vi "parseILC.vi"(8 "error in (no error)":errorcluster, 9 "Func":u8=255, 10 "ModbusBuffer in":refnum<class "ModbusBuffer.lvclass">, 11 "ILC in":refnum<class "ILC.lvclass">) -> (0 "error out":errorcluster, 1 "ParseSuccessful":bool, 2 "ModbusBuffer out":refnum<class "ModbusBuffer.lvclass">, 3 "ILC out":refnum<class "ILC.lvclass">)   [LabVIEW 2016, in "RTILC.lvlib" / "ILC.lvclass"]
uses:
  ILC.lvclass
  Common_RT_Modbus/ModbusBuffer/ModbusBuffer.lvclass
  Common_RT_Modbus/ModbusBuffer/ModbusBuffer.lvclass/ModbusBuffer.ctl
  ILC.lvclass/ILC.ctl
  Common_RT_Modbus/ModbusBuffer/calculateCRC.vi
  Common_RT_Modbus/ModbusBuffer/readCRC.vi
  Common_RT_Modbus/ModbusBuffer/readTimestamp.vi
  Common_RT_Modbus/ModbusBuffer/readEndOfFrame.vi
  Common_RT_Modbus/ModbusBuffer/readU48.vi
  Common_RT_Modbus/ModbusBuffer/readString.vi
  Common_RT_Modbus/ModbusBuffer/readU16.vi
  Common_RT_Modbus/ModbusBuffer/readSGL.vi
  Common_RT_Modbus/ModbusBuffer/readInstructionByte.vi
  Common_RT_Modbus/ModbusBuffer/readTimestampByte.vi
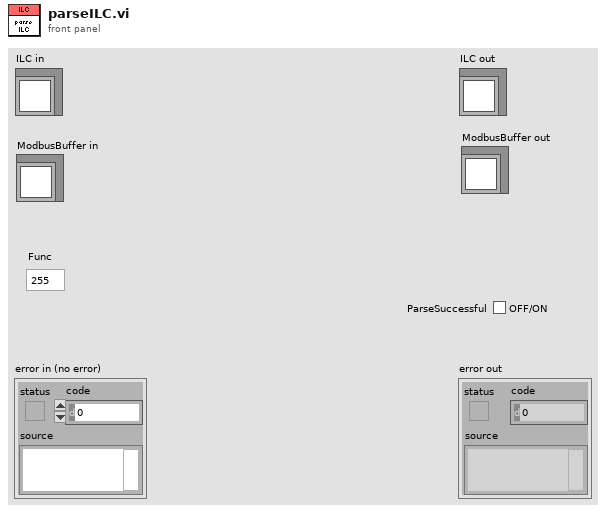
[diagram p1: front panel]
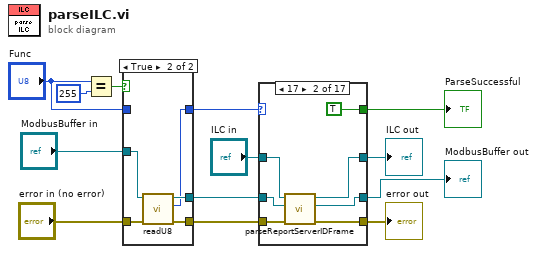
[diagram p0: block diagram]
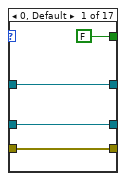
[diagram p3: hidden frame]
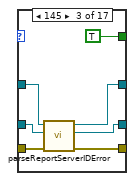
[diagram p4: hidden frame]
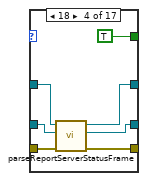
[diagram p5: hidden frame]
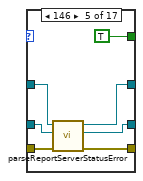
[diagram p6: hidden frame]
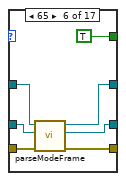
[diagram p7: hidden frame]
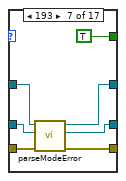
[diagram p8: hidden frame]
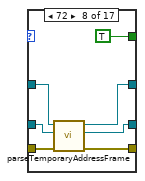
[diagram p9: hidden frame]
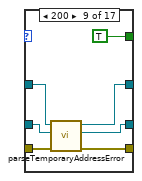
[diagram p10: hidden frame]
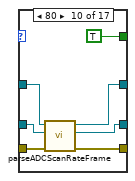
[diagram p11: hidden frame]
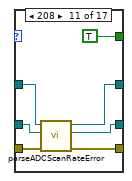
[diagram p12: hidden frame]
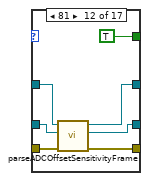
[diagram p13: hidden frame]
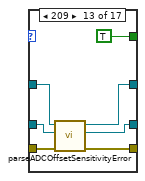
[diagram p14: hidden frame]
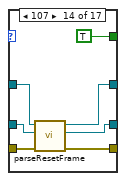
[diagram p15: hidden frame]
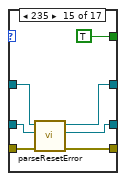
[diagram p16: hidden frame]
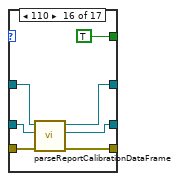
[diagram p17: hidden frame]
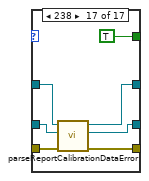
[diagram p18: hidden frame]
diagram:
  n1 = Equal?(x="Func", y=u8 255) -> (x = y?=w2:bool)
  n2 = case shown="True" w2 {
    tunnel: "ModbusBuffer in" -> [w15 w21]
    tunnel: [w15 w20] -> w9
    tunnel: [w16 w19] -> w8
    tunnel: [w14 w18] -> w7
    tunnel: "error in (no error)" -> [w14 w17]
    tunnel: "Func" -> [w16 _]
    frame False {
    }
    frame True {
      n3 = call "readU8.vi"("error in (no error)"=w17, "ModbusBuffer in"=w21) -> ("error out"=w18:errorcluster, "Output"=w19:u8, "ModbusBuffer out"=w20:refnum<class "ModbusBuffer.lvclass">)  [unwired: 7 in]
    }
  }
  n4 = case shown="17" w8 {
    tunnel: [FALSE TRUE TRUE TRUE TRUE TRUE TRUE TRUE TRUE TRUE TRUE TRUE TRUE TRUE TRUE TRUE TRUE] -> w13
    tunnel: "ILC in" -> [w24 w32 w39 w46 w53 w59 w67 w74 w81 w88 w95 w102 w109 w116 w123 w130 w137]
    tunnel: w9 -> [w23 w31 w38 w44 w51 w60 w66 w73 w80 w87 w94 w101 w108 w115 w122 w129 w136]
    tunnel: [w24 w30 w37 w45 w52 w58 w65 w72 w79 w86 w93 w100 w107 w114 w121 w128 w135] -> w11
    tunnel: [w23 w28 w35 w42 w49 w56 w63 w70 w77 w84 w91 w98 w105 w112 w119 w126 w133] -> w4
    tunnel: w7 -> [w22 w27 w33 w41 w48 w55 w62 w69 w76 w83 w90 w97 w104 w111 w118 w125 w132]
    tunnel: [w22 w26 w34 w40 w47 w54 w61 w68 w75 w82 w89 w96 w103 w110 w117 w124 w131] -> w5
    frame 0, Default {
    }
    frame 17 {
      n5 = call "parseReportServerIDFrame.vi"("error in (no error)"=w27, "ModbusBuffer in"=w31, "ILC in"=w32) -> ("error out"=w26:errorcluster, "ModbusBuffer out"=w28:refnum<class "ModbusBuffer.lvclass">, "ILC out"=w30:refnum<class "ILC.lvclass">)  [unwired: 6 in]
    }
    frame 145 {
      n6 = call "parseReportServerIDError.vi"("error in (no error)"=w33, "ModbusBuffer in"=w38, "ILC in"=w39) -> ("error out"=w34:errorcluster, "ModbusBuffer out"=w35:refnum<class "ModbusBuffer.lvclass">, "ILC out"=w37:refnum<class "ILC.lvclass">)  [unwired: 6 in]
    }
    frame 18 {
      n7 = call "parseReportServerStatusFrame.vi"("error in (no error)"=w41, "ModbusBuffer in"=w44, "ILC in"=w46) -> ("error out"=w40:errorcluster, "ModbusBuffer out"=w42:refnum<class "ModbusBuffer.lvclass">, "ILC out"=w45:refnum<class "ILC.lvclass">)  [unwired: 6 in]
    }
    frame 146 {
      n8 = call "parseReportServerStatusError.vi"("error in (no error)"=w48, "ModbusBuffer in"=w51, "ILC in"=w53) -> ("error out"=w47:errorcluster, "ModbusBuffer out"=w49:refnum<class "ModbusBuffer.lvclass">, "ILC out"=w52:refnum<class "ILC.lvclass">)  [unwired: 6 in]
    }
    frame 65 {
      n9 = call "parseModeFrame.vi"("error in (no error)"=w55, "ModbusBuffer in"=w60, "ILC in"=w59) -> ("error out"=w54:errorcluster, "ModbusBuffer out"=w56:refnum<class "ModbusBuffer.lvclass">, "ILC out"=w58:refnum<class "ILC.lvclass">)  [unwired: 6 in]
    }
    frame 193 {
      n10 = call "parseModeError.vi"("error in (no error)"=w62, "ModbusBuffer in"=w66, "ILC in"=w67) -> ("error out"=w61:errorcluster, "ModbusBuffer out"=w63:refnum<class "ModbusBuffer.lvclass">, "ILC out"=w65:refnum<class "ILC.lvclass">)  [unwired: 6 in]
    }
    frame 72 {
      n11 = call "parseTemporaryAddressFrame.vi"("error in (no error)"=w69, "ModbusBuffer in"=w73, "ILC in"=w74) -> ("error out"=w68:errorcluster, "ModbusBuffer out"=w70:refnum<class "ModbusBuffer.lvclass">, "ILC out"=w72:refnum<class "ILC.lvclass">)  [unwired: 6 in]
    }
    frame 200 {
      n12 = call "parseTemporaryAddressError.vi"("error in (no error)"=w76, "ModbusBuffer in"=w80, "ILC in"=w81) -> ("error out"=w75:errorcluster, "ModbusBuffer out"=w77:refnum<class "ModbusBuffer.lvclass">, "ILC out"=w79:refnum<class "ILC.lvclass">)  [unwired: 6 in]
    }
    frame 80 {
      n13 = call "parseADCScanRateFrame.vi"("error in (no error)"=w83, "ModbusBuffer in"=w87, "ILC in"=w88) -> ("error out"=w82:errorcluster, "ModbusBuffer out"=w84:refnum<class "ModbusBuffer.lvclass">, "ILC out"=w86:refnum<class "ILC.lvclass">)  [unwired: 6 in]
    }
    frame 208 {
      n14 = call "parseADCScanRateError.vi"("error in (no error)"=w90, "ModbusBuffer in"=w94, "ILC in"=w95) -> ("error out"=w89:errorcluster, "ModbusBuffer out"=w91:refnum<class "ModbusBuffer.lvclass">, "ILC out"=w93:refnum<class "ILC.lvclass">)  [unwired: 6 in]
    }
    frame 81 {
      n15 = call "parseADCOffsetSensitivityFrame.vi"("error in (no error)"=w97, "ModbusBuffer in"=w101, "ILC in"=w102) -> ("error out"=w96:errorcluster, "ModbusBuffer out"=w98:refnum<class "ModbusBuffer.lvclass">, "ILC out"=w100:refnum<class "ILC.lvclass">)  [unwired: 6 in]
    }
    frame 209 {
      n16 = call "parseADCOffsetSensitivityError.vi"("error in (no error)"=w104, "ModbusBuffer in"=w108, "ILC in"=w109) -> ("error out"=w103:errorcluster, "ModbusBuffer out"=w105:refnum<class "ModbusBuffer.lvclass">, "ILC out"=w107:refnum<class "ILC.lvclass">)  [unwired: 6 in]
    }
    frame 107 {
      n17 = call "parseResetFrame.vi"("error in (no error)"=w111, "ModbusBuffer in"=w115, "ILC in"=w116) -> ("error out"=w110:errorcluster, "ModbusBuffer out"=w112:refnum<class "ModbusBuffer.lvclass">, "ILC out"=w114:refnum<class "ILC.lvclass">)  [unwired: 6 in]
    }
    frame 235 {
      n18 = call "parseResetError.vi"("error in (no error)"=w118, "ModbusBuffer in"=w122, "ILC in"=w123) -> ("error out"=w117:errorcluster, "ModbusBuffer out"=w119:refnum<class "ModbusBuffer.lvclass">, "ILC out"=w121:refnum<class "ILC.lvclass">)  [unwired: 6 in]
    }
    frame 110 {
      n19 = call "parseReportCalibrationDataFrame.vi"("error in (no error)"=w125, "ModbusBuffer in"=w129, "ILC in"=w130) -> ("error out"=w124:errorcluster, "ModbusBuffer out"=w126:refnum<class "ModbusBuffer.lvclass">, "ILC out"=w128:refnum<class "ILC.lvclass">)  [unwired: 6 in]
    }
    frame 238 {
      n20 = call "parseReportCalibrationDataError.vi"("error in (no error)"=w132, "ModbusBuffer in"=w136, "ILC in"=w137) -> ("error out"=w131:errorcluster, "ModbusBuffer out"=w133:refnum<class "ModbusBuffer.lvclass">, "ILC out"=w135:refnum<class "ILC.lvclass">)  [unwired: 6 in]
    }
  }
  "error out" <- w5
  "ILC out" <- w11
  "ParseSuccessful" <- w13
  "ModbusBuffer out" <- w4
